vi "Call Revert to Scan Mode.vi"(8 "error in":errorcluster, 10 "Target IP Address":string, 11 "Slave Ref":string) -> (0 "error out":errorcluster)   [LabVIEW 2020, in "SEECD System Explorer.lvlib"]
uses:
  SEECD System Explorer.lvlib
  f4c09cb3-a82b-42f6-9055-d4148a851ace.vi
  00f8f119-917a-4c23-8807-b8d445e03b72.vi
  f4c09cb3-a82b-42f6-9055-d4148a851ace.vi/ff40df25-0e41-4205-825d-56c19dc320b6.vi
  00f8f119-917a-4c23-8807-b8d445e03b72.vi/ff40df25-0e41-4205-825d-56c19dc320b6.vi
  <vilib>/Utility/Debug Log/Display.vi
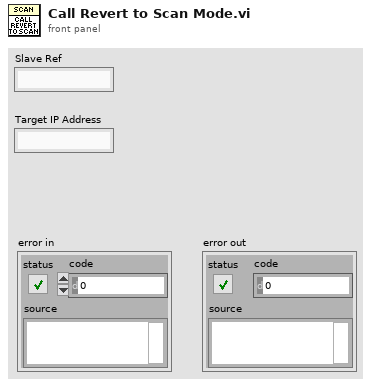
[diagram p1: front panel]
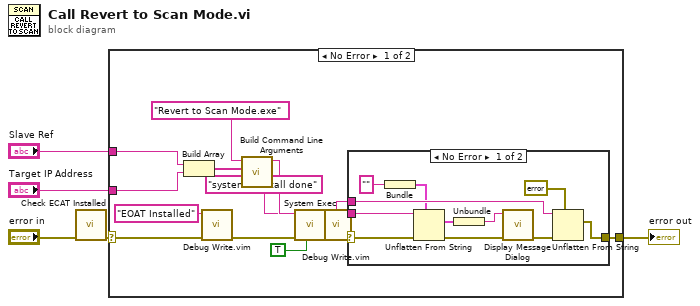
[diagram p0: block diagram]
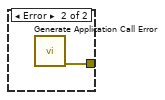
[diagram p2: hidden frame]
diagram:
  n1 = call "Check ECAT Installed.vi"("error in"="error in") -> ("error out"=w1:errorcluster)  [unwired: 10 in]
  n2 = case shown="No Error" w1 {
    selector: w1 -> [w20 w33]
    tunnel: [w18 w33] -> w3
    tunnel: "Slave Ref" -> [w14 _]
    tunnel: "Target IP Address" -> [w13 _]
    frame No Error {
      n3 = Build Array(w14, w13) -> (w12:string[])
      n4 = call "Debug Write.vim"("error in (no error)"=w20, "value"="EOAT Installed") -> ("error out"=w9:errorcluster)  [unwired: 9 in]
      n5 = call "Build Command Line Arguments.vi"("Arguments"=w12, "Executable File Name"="Revert to Scan Mode.exe" ("name or relative path")) -> ("Command Line"=w11:string)  [unwired: 9 in]
      n6 = call <vilib>:"System Exec.vi"("run minimized? (F)"=TRUE, "error in (no error)"=w9, "command line"=w11) -> ("error out"=w19:errorcluster, "standard error"=w17:string, "standard output"=w10:string)  [unwired: 5 in, 1 out]
      n7 = call "Debug Write.vim"("error in (no error)"=w19, "value"="system exe call done") -> ("error out"=w7:errorcluster)  [unwired: 9 in]
      n8 = case shown="No Error" w7 {
        selector: w7 -> [w27 _]
        tunnel: [w30 w32] -> w18
        tunnel: w17 -> [w29 _]
        tunnel: w10 -> [w24 _]
        frame No Error {
          n9 = Bundle("") -> (w25:cluster{string})  [unwired: 1 in]
          n10 = Unflatten From String(type=w25, binary string=w24, error in (no error)=w27) -> (value=w22:cluster{string}, error out=w26:errorcluster)  [unwired: 2 in, 1 out]
          n11 = Unbundle(w22) -> (w21:string)
          n12 = call "Display Message Dialog.vi"("error in"=w26, "Message to display"=w21) -> ("error out"=w28:errorcluster)  [unwired: 9 in]
          n13 = Unflatten From String(type=errorcluster {"status"=FALSE, "code"=0, "source"=""} ("error in (no error)"), binary string=w29, error in (no error)=w28) -> (value=w30:errorcluster)  [unwired: 2 in, 2 out]
        }
        frame Error {
          n14 = call "Generate Application Call Error.vi"() -> ("error out"=w32:errorcluster)  [unwired: 11 in]
        }
      }
    }
    frame Error {
    }
  }
  "error out" <- w3
